vi "test--save-for-previous.vi"() -> ()   [LabVIEW 2021]
uses:
  project/_button-editor/TSC Button Editor.lvclass
panel:
  out "error out 2":errorcluster
  in  "Save For:":string(combo)="24.0"
  out "Warnings":string
  out "error out":errorcluster
  in  "Target Version":string
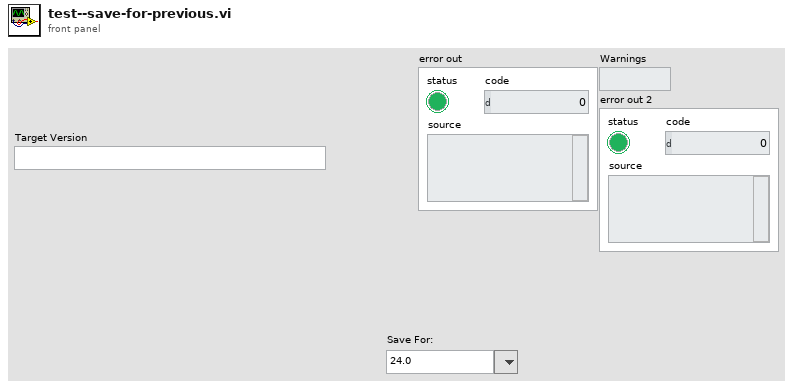
[diagram p1: front panel]
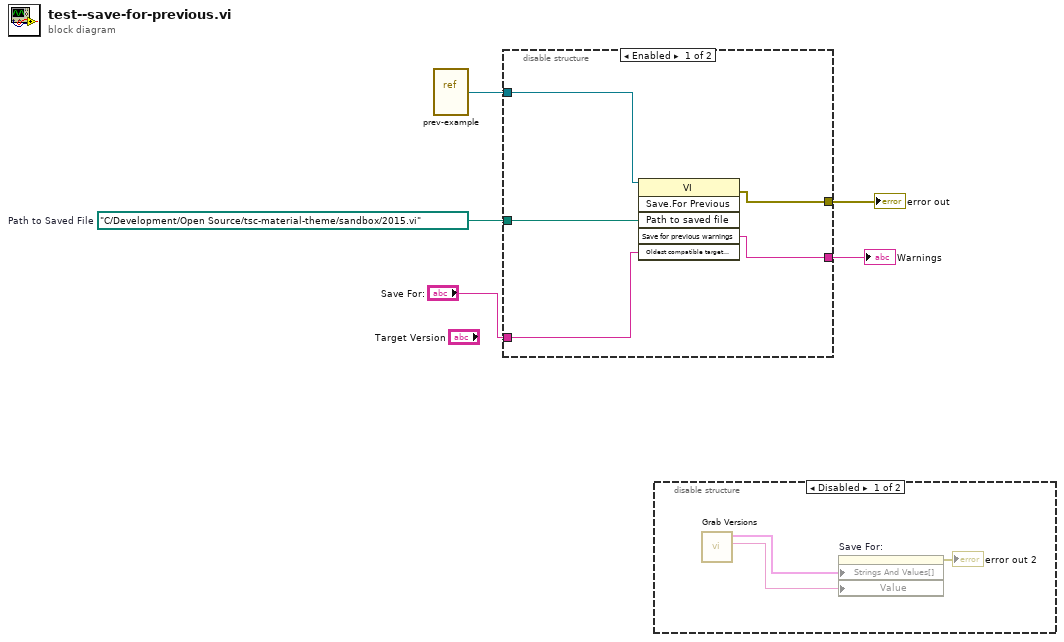
[diagram p0: block diagram]
diagram:
  w3 = path "C:/Development/Open Source/tsc-material-theme/sandbox/2015.vi"  # Path to Saved File
  n1 = vi-ref "prev-example.vi"() -> (w2:refnum<vi>)
  n2 = disable-structure shown="Enabled" {
    disable-tunnel: "Save For:" -> [w10 _]
    disable-tunnel: [w9 _] -> w5
    disable-tunnel: [w8 _] -> w4
    disable-tunnel: w3 -> [w7 _]
    disable-tunnel: w2 -> [w6 _]
    frame Enabled {
      n3 = invoke class="VI" method="Save.For Previous"(reference=w6, "Path to saved file"=w7, "Oldest compatible target version"=w10) -> (error out=w9:errorcluster, "Save for previous warnings"=w8:string)  [unwired: 3 in, 4 out]
    }
    frame Disabled {
    }
  }
  "error out" <- w5
  "Warnings" <- w4
  n4 = disable-structure shown="Disabled" {
    frame Disabled {
      n5 = call "Grab Versions.vi"() -> ("Selection"=w11:string, "Strings and Values"=w12:cluster{"string":string, "value":string}[])  [unwired: 10 in]
      n6 = property on="Save For:" class="CmbBox"("Strings And Values[]"=w12, "Value"=w11) -> (error out=→"error out 2":errorcluster)  [unwired: 2 in, 1 out]
    }
    frame Enabled {
    }
  }
